vi "dialog_box (2).vi"(10 "INPUT":string) -> (3 "Boolean":bool=TRUE)   [LabVIEW 2020]
panel:
  out "String":string
  in  "NO":bool
  in  "YES":bool
  # "MSG BOX"
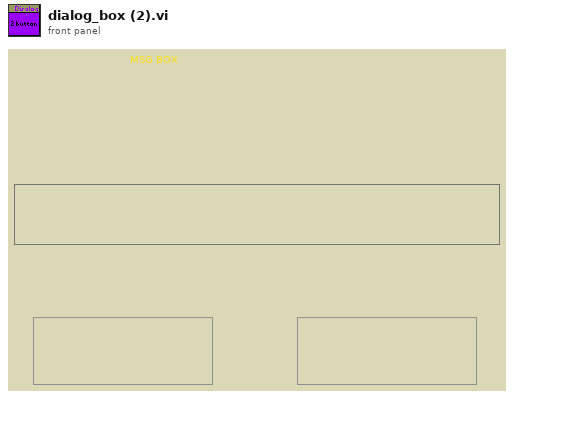
[diagram p1: front panel]
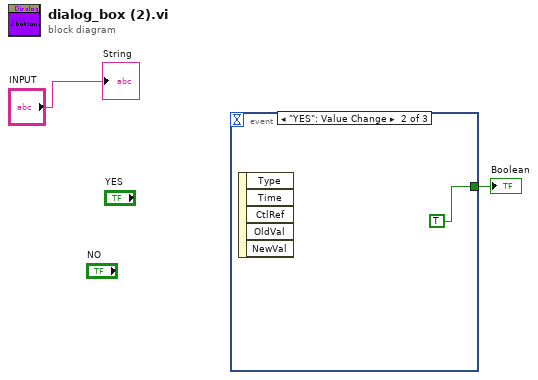
[diagram p0: block diagram]
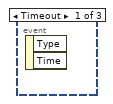
[diagram p2: hidden frame]
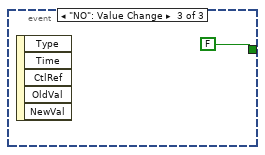
[diagram p3: hidden frame]
diagram:
  n1 = event shown="[1] \"YES\": Value Change" {
    selector: _ -> [_ _ _]
    dyn-events: _ -> [_ _ _]
    timeout: _ -> [_ _ _]
    tunnel: [_ TRUE FALSE] -> w2
    event Timeout {
      n2 = event-data() -> ()  [unwired: 1 in, 2 out]
    }
    event "YES": Value Change {
      n3 = event-data() -> ()  [unwired: 1 in, 5 out]
    }
    event "NO": Value Change {
      n4 = event-data() -> ()  [unwired: 1 in, 5 out]
    }
  }
  "Boolean" <- w2
  "String" <- "INPUT"
